vi "Wrapper.vi"(0 "measurement configuration":T1={"pin_name"="Lorem ipsum dolor sit", "Option String (\"\")"="", "Connection Specification (\"\")"="", "Initialization Behavior"=enum."Auto"}, 11 "error in":errorcluster) -> (4 "measurement results":T3, 15 "error out":errorcluster)   [LabVIEW 2021, in "SimpleSwitchConnect.lvlib"]
uses:
  SimpleSwitchConnect.lvlib
  MeasurementCore/SimpleSwitch/SimpleSwitch_Reusables.lvlib
  Measurement Results.ctl
  Measurement Configuration.ctl
  SimpleSwitch UI/Initialization Behavior.ctl
  SimpleSwitch UI/SimpleSwitchConnect UI.lvlib
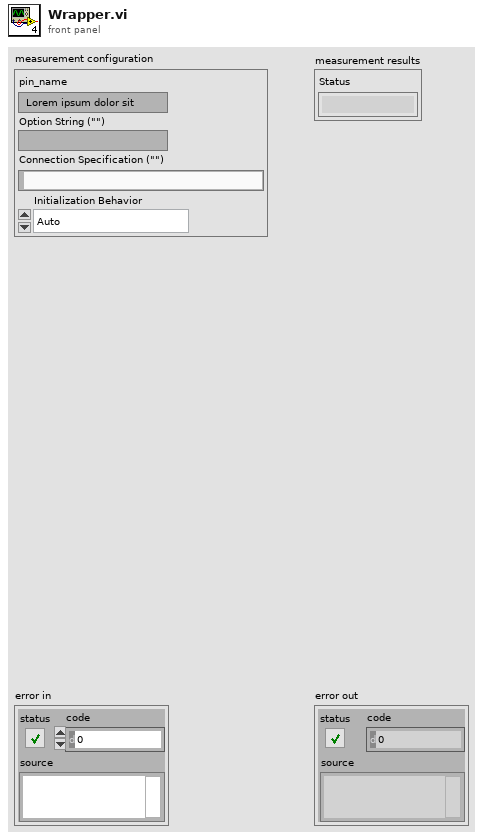
[diagram p1: front panel]
types:
  T1 = typedef "SimpleSwitchConnect.lvlib/Measurement Configuration.ctl" = cluster{"pin_name":string, "Option String (\"\")":string, "Connection Specification (\"\")":string, "Initialization Behavior":T2}
  T2 = typedef "SimpleSwitchConnect UI.lvlib/Initialization Behavior.ctl" = enum32{"Auto", "Initialize and Close", "Attach and Detach", "Initialize and Detach", "Attach and Close"}
  T3 = typedef "SimpleSwitchConnect.lvlib/Measurement Results.ctl" = cluster{"Status":string}
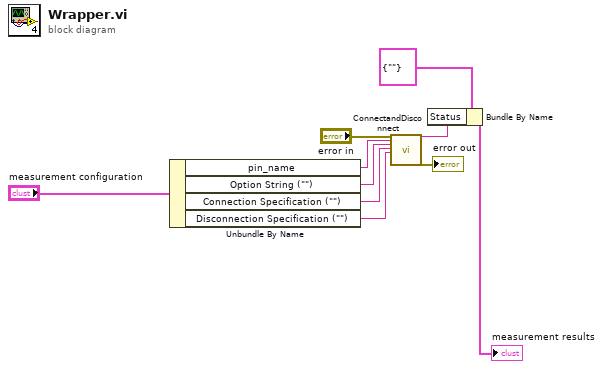
[diagram p0: block diagram]
diagram:
  n1 = Unbundle By Name("measurement configuration") -> ("pin_name"=w9:string, "Option String (\"\")"=w8:string, "Connection Specification (\"\")"=w7:string, "Disconnection Specification (\"\")"=w6:string)
  n2 = call "ConnectandDisconnect.vi"("error in"="error in", "Virtual Device Name"=w9, "Option String (\"\")"=w8, "Connection Specification (\"\")"=w7, "Disconnection Specification (\"\")"=w6) -> ("Status"=w3:string, "error out"=→"error out":errorcluster)  [unwired: 21 in]
  n3 = Bundle By Name(cluster=T3 {"Status"=""} ("measurement results"), "Status"=w3) -> (→"measurement results":T3)
